vi "is_empy_timestamp.vi"(2 "time stamp":timestamp) -> (7 "is empty?":bool)   [LabVIEW 2015]
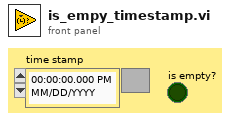
[diagram p1: front panel]
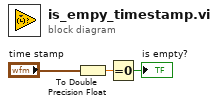
[diagram p0: block diagram]
diagram:
  n1 = To Double Precision Float(number="time stamp") -> (double precision float=w2:dbl)
  n2 = Equal To 0?(x=w2) -> (x = 0?=→"is empty?":bool)
